vi "LINC Set Item Configuration.vi"(4 "value":string, 6 "config type":T1, 7 "item name":string, 8 "error in (no error)":errorcluster, 9 "packet name":string, 10 "type":enum16{"CMD", "TLM"}(ring), 11 "LINC session":refnum<class "LINC.lvclass">) -> (0 "error out":errorcluster, 3 "dup LINC session":refnum<class "LINC.lvclass">)   [LabVIEW 2018, in "STEPkgDriver_LINC.lvlib" / "LINC.lvclass"]
uses:
  LINC.lvclass
  LINC Global Mode.ctl
  STEPkgDriver_LINC.lvlib
  LINC Config Type.ctl
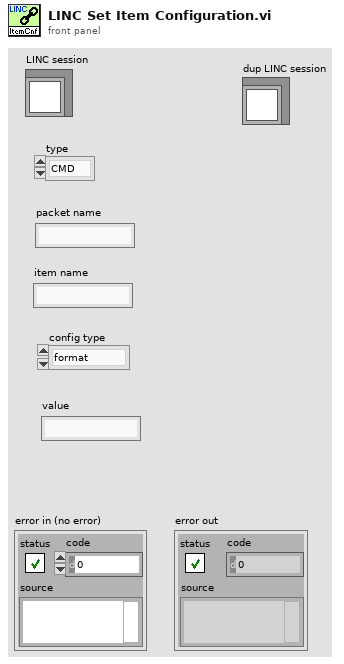
[diagram p1: front panel]
types:
  T1 = typedef "STEPkgDriver_LINC.lvlib/LINC Config Type.ctl" = enum16{"format", "unit", "description", "max", "min", "default"}
  T2 = typedef "STEPkgDriver_LINC.lvlib/LINC Global Mode.ctl" = enum16{"INIT", "CLEAR", "ADD_PKT_HDR", "ADD_PKT", "GET_PKT_NAMES", "GET_PKT_DESC", "GET_PKT_HDR", "GET_PKT", "SET_PKT", "SET_DATA", "SIM_EN", "SIM_DS"}
  T3 = typedef "STEPkgDriver_LINC.lvlib/LINC Format Prototype.ctl" = cluster{"type":string, "bit offset":i32, "bit size":i32, "format":string, "unit":string, "description":string, "state values":i64[], "states":string[], "max":string, "min":string, "default":string, "array":bool, "bit element size":i32, "poly bound":dbl[], "poly scale":cluster{"coefficients":dbl[]}[], "labview size":i32, "simulate":bool, "ID":bool, "required":bool}
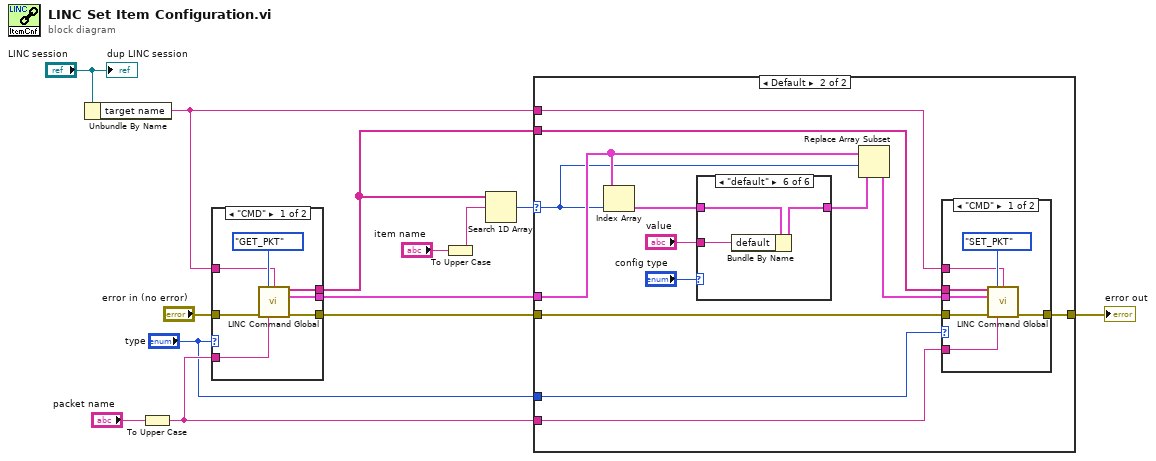
[diagram p0: block diagram]
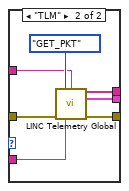
[diagram p2: hidden frame]
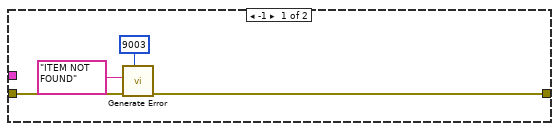
[diagram p3: hidden frame]
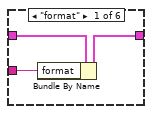
[diagram p4: hidden frame]
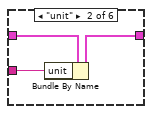
[diagram p5: hidden frame]
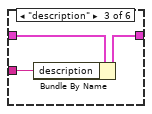
[diagram p6: hidden frame]
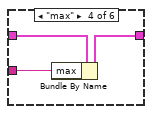
[diagram p7: hidden frame]
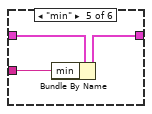
[diagram p8: hidden frame]
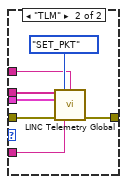
[diagram p9: hidden frame]
diagram:
  n1 = Unbundle By Name("LINC session") -> ("target name"=w3:string)
  n2 = To Upper Case(1:"packet name") -> (0:w2:string)
  n3 = case shown="\"CMD\"" "type" {
    tunnel: "error in (no error)" -> [w19 w27]
    tunnel: [w18 w25] -> w9
    tunnel: [w14 w24] -> w5
    tunnel: [w15 w23] -> w4
    tunnel: w3 -> [w17 w22]
    tunnel: w2 -> [w16 w21]
    frame "CMD" {
      n4 = call "LINC Command Global.vi"("mode"=LINC_Global_Mode."GET_PKT", "target name"=w17, "error in (no error)"=w19, "packet name"=w16) -> ("values out"=w15:string[], "item formats out"=w14:T3[], "error out"=w18:errorcluster)  [unwired: 7 in, 2 out]
    }
    frame "TLM" {
      n5 = call "LINC Telemetry Global.vi"("mode"=LINC_Global_Mode."GET_PKT", "target name"=w22, "error in (no error)"=w27, "packet name"=w21) -> ("values out"=w23:string[], "item formats out"=w24:T3[], "error out"=w25:errorcluster)  [unwired: 7 in, 2 out]
    }
  }
  n6 = To Upper Case(1:"item name") -> (0:w7:string)
  n7 = Search 1D Array(1D array=w4, element=w7) -> (index of element=w6:i32)  [unwired: 1 in]
  n8 = case shown="Default" w6 {
    selector: w6 -> [_ w40]
    tunnel: [w30 w44] -> w12
    tunnel: w9 -> [w31 w43]
    tunnel: w3 -> [_ w37]
    tunnel: w2 -> [_ w36]
    tunnel: w5 -> [_ w41]
    tunnel: w4 -> [_ w38]
    tunnel: "type" -> [_ w35]
    frame -1 {
      n9 = call "Generate Error.vi"("error code (-1301)"=9003, "error in"=w31, "description"="ITEM NOT FOUND") -> ("error out"=w30:errorcluster)  [unwired: 8 in]
    }
    frame Default {
      n10 = Index Array(array=w41, index=w40) -> (element=w42:T3)
      n11 = case shown="\"default\"" "config type" {
        tunnel: w42 -> [w47 w50 w53 w56 w59 w62]
        tunnel: [w46 w49 w52 w55 w58 w61] -> w34
        tunnel: "value" -> [w45 w48 w51 w54 w57 w60]
        frame "format" {
          n12 = Bundle By Name(cluster=w47, "format"=w45) -> (w46:T3)
        }
        frame "unit" {
          n13 = Bundle By Name(cluster=w50, "unit"=w48) -> (w49:T3)
        }
        frame "description" {
          n14 = Bundle By Name(cluster=w53, "description"=w51) -> (w52:T3)
        }
        frame "max" {
          n15 = Bundle By Name(cluster=w56, "max"=w54) -> (w55:T3)
        }
        frame "min" {
          n16 = Bundle By Name(cluster=w59, "min"=w57) -> (w58:T3)
        }
        frame "default" {
          n17 = Bundle By Name(cluster=w62, "default"=w60) -> (w61:T3)
        }
      }
      n18 = Replace Array Subset(array=w41, new element=w34, index=w40) -> (w39:T3[])
      n19 = case shown="\"CMD\"" w35 {
        tunnel: [w68 w75] -> w44
        tunnel: w43 -> [w67 w74]
        tunnel: w39 -> [w66 w73]
        tunnel: w38 -> [w65 w72]
        tunnel: w37 -> [w64 w71]
        tunnel: w36 -> [w63 w70]
        frame "CMD" {
          n20 = call "LINC Command Global.vi"("item names in"=w65, "mode"=LINC_Global_Mode."SET_PKT", "target name"=w64, "item formats in"=w66, "error in (no error)"=w67, "packet name"=w63) -> ("error out"=w68:errorcluster)  [unwired: 5 in, 4 out]
        }
        frame "TLM" {
          n21 = call "LINC Telemetry Global.vi"("item names in"=w72, "mode"=LINC_Global_Mode."SET_PKT", "target name"=w71, "item formats in"=w73, "error in (no error)"=w74, "packet name"=w70) -> ("error out"=w75:errorcluster)  [unwired: 5 in, 4 out]
        }
      }
    }
  }
  "error out" <- w12
  "dup LINC session" <- "LINC session"
